vi "Return DeviceComms.vi"(8 "error in (no error)":errorcluster, 10 "DeviceComms":refnum<class "DeviceComms.lvclass">, 11 "Session in":refnum<class "Session.lvclass">) -> (0 "error out":errorcluster, 3 "Session out":refnum<class "Session.lvclass">)   [LabVIEW 2020, in "CTI.lvlib" / "Session.lvclass"]
doc: "This VI needs to be called after every call of <b>Acquire DeviceComms.vi</b> for proper operation of the session otherwise future attempts to interact with a device will fail. Returning the DeviceComms instance allows any parallel operations that are waiting to begin."
uses:
  Session.lvclass
  DeviceComms/DeviceComms.lvclass
  Session.lvclass/Session.ctl
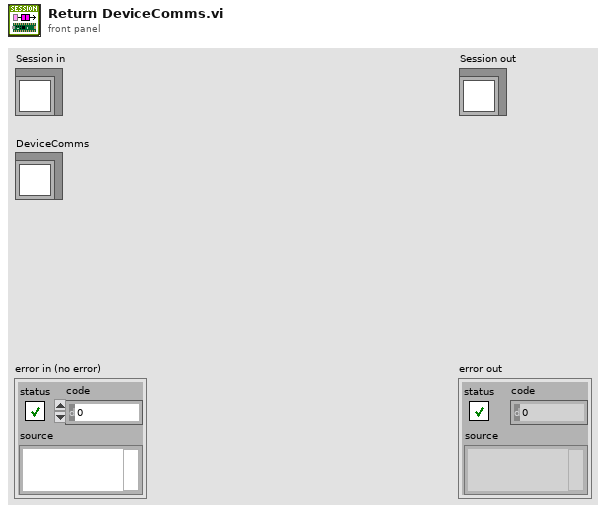
[diagram p1: front panel]
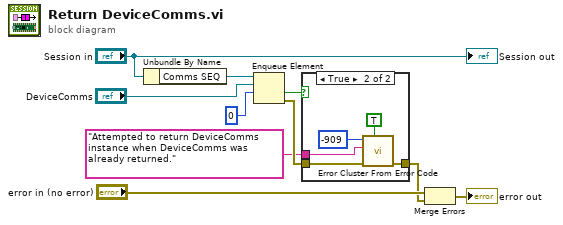
[diagram p0: block diagram]
diagram:
  n1 = Unbundle By Name("Session in") -> ("Comms SEQ"=w9:refnum<queue>)
  n2 = Enqueue Element(queue=w9, element="DeviceComms", timeout in ms (-1)=0) -> (timed out?=w3:bool, error out=w4:errorcluster)  [unwired: 1 in, 1 out]
  n3 = case shown="True" w3 {
    tunnel: w4 -> [w11 w16]
    tunnel: [w11 w15] -> w2
    tunnel: "Attempted to return DeviceComms instance when DeviceComms was already returned." -> [_ w12]
    frame False {
    }
    frame True {
      n4 = call <vilib>:"Error Cluster From Error Code.vi"("show call chain? (False)"=TRUE, "error in (no error)"=w16, "error message (\"\")"=w12, "error code (0)"=-909) -> ("error out"=w15:errorcluster)  [unwired: 5 in]
    }
  }
  n5 = Merge Errors("error in (no error)", w2) -> (→"error out":errorcluster)
  "Session out" <- "Session in"
